vi "Scale Intensity Plot.vi"(7 "Dimensions":i32[](array[numeric]), 8 "error in (no error)":errorcluster, 9 "Y Range":cluster{"Min":dbl, "Max":dbl, "Increment":dbl}, 10 "X Range":cluster{"Min":dbl, "Max":dbl, "Increment":dbl}, 11 "IntGraph Refnum":refnum<vi>) -> (0 "error out":errorcluster, 3 "IntGraph Refnum out":refnum<vi>)   [LabVIEW 2010]
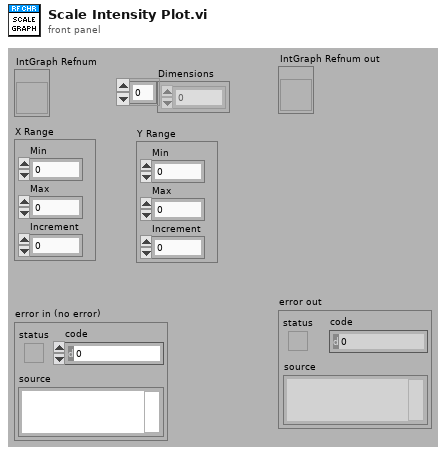
[diagram p1: front panel]
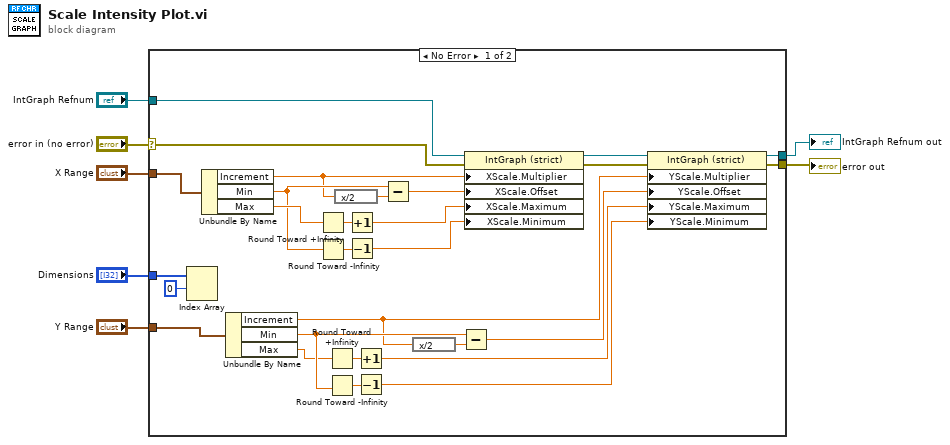
[diagram p0: block diagram]
diagram:
  n1 = case shown="No Error" "error in (no error)" {
    selector: "error in (no error)" -> [w26 w37]
    tunnel: "Y Range" -> [w35 _]
    tunnel: "X Range" -> [w34 _]
    tunnel: "IntGraph Refnum" -> [w33 w36]
    tunnel: "Dimensions" -> [w31 _]
    tunnel: [w28 w37] -> w3
    tunnel: [w27 w36] -> w2
    frame No Error {
      n2 = Index Array(array=w31, index #1=0 ("index")) -> ()  [unwired: 1 in, 2 out]
      n3 = Unbundle By Name(w34) -> ("Increment"=w8:dbl, "Min"=w10:dbl, "Max"=w12:dbl)
      n4 = Unbundle By Name(w35) -> ("Increment"=w16:dbl, "Min"=w17:dbl, "Max"=w13:dbl)
      n5 = Round Toward +Infinity(x=w12) -> (ceil(x): smallest int >= x=w25:dbl)
      n6 = Round Toward -Infinity(1:w10) -> (0:w23:dbl)
      n7 = Round Toward +Infinity(x=w13) -> (ceil(x): smallest int >= x=w20:dbl)
      n8 = Round Toward -Infinity(1:w17) -> (0:w21:dbl)
      n9 = expression code="x/2"(w8) -> (w11:dbl)
      n10 = Increment(x=w25) -> (x+1=w24:dbl)
      n11 = Decrement(x=w23) -> (x-1=w22:dbl)
      n12 = Increment(x=w20) -> (x+1=w19:dbl)
      n13 = Decrement(x=w21) -> (x-1=w18:dbl)
      n14 = Subtract(x=w10, y=w11) -> (x-y=w9:dbl)
      n15 = expression code="x/2"(w16) -> (w15:dbl)
      n16 = Subtract(x=w17, y=w15) -> (x-y=w14:dbl)
      n17 = property on="Property Node" class="IntGraph (strict)"(reference=w33, error in=w26, "XScale.Multiplier"=w8, "XScale.Offset"=w9, "XScale.Maximum"=w24, "XScale.Minimum"=w22) -> (reference out=w30:refnum<vi>, error out=w29:errorcluster)
      n18 = property on="Property Node" class="IntGraph (strict)"(reference=w30, error in=w29, "YScale.Multiplier"=w16, "YScale.Offset"=w14, "YScale.Maximum"=w19, "YScale.Minimum"=w18) -> (reference out=w27:refnum<vi>, error out=w28:errorcluster)
    }
    frame Error {
    }
  }
  "error out" <- w3
  "IntGraph Refnum out" <- w2
